vi "shuffled array 1d.vi"() -> ()   [LabVIEW 2025]
uses:
  7d14f3a8-1a65-44ef-a868-b4e55e2935ab.vi
panel:
  out "reverse array":dbl[](array[numeric])
  in  "input array":dbl[](array[numeric])
  out "shuffled array":dbl[](array[numeric])
  in  "Array":dbl[](array[numeric])
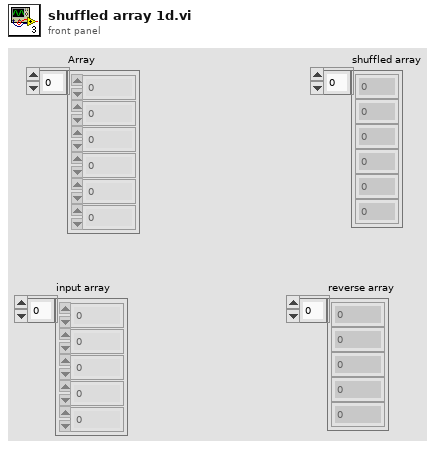
[diagram p1: front panel]
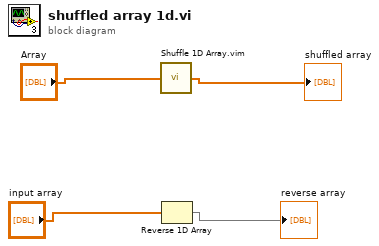
[diagram p0: block diagram]
diagram:
  n1 = call "Shuffle 1D Array.vim"("array"="Array") -> ("shuffled array"=→"shuffled array":dbl[])  [unwired: 4 in]
  n2 = Reverse 1D Array(array="input array") -> (reversed array=→"reverse array":dbl[])
